vi "Get Device.vi"(6 "error in":errorcluster, 9 "String":string) -> (0 "error out 2":errorcluster, 2 "element":string, 3 "substring":string)   [LabVIEW 2013]
uses:
  <vilib>/regexp/Match Regular Expression.xnode
panel:
  out "Device Name":string
  out "Numeric":i32
  out "Sorted List":string[](array[string])
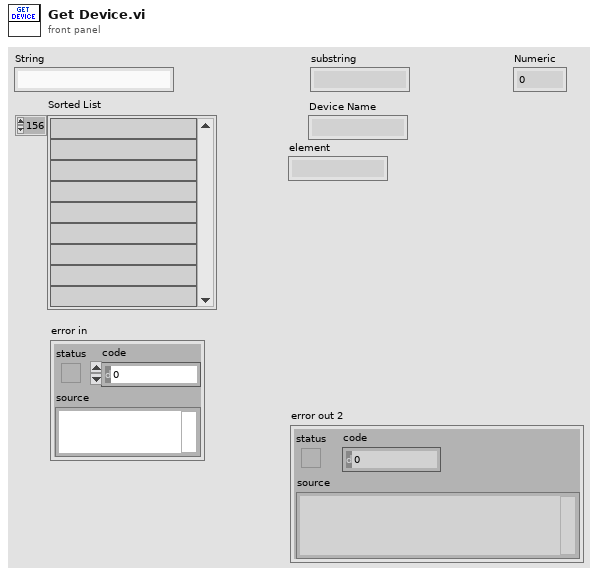
[diagram p1: front panel]
types:
  T1 = typedef "mysql_authentication.ctl" = cluster{"User":string, "Password":string, "Database":string}
  T2 = cluster{"Port":u16, "IP Address":string, "Authentication":T1}
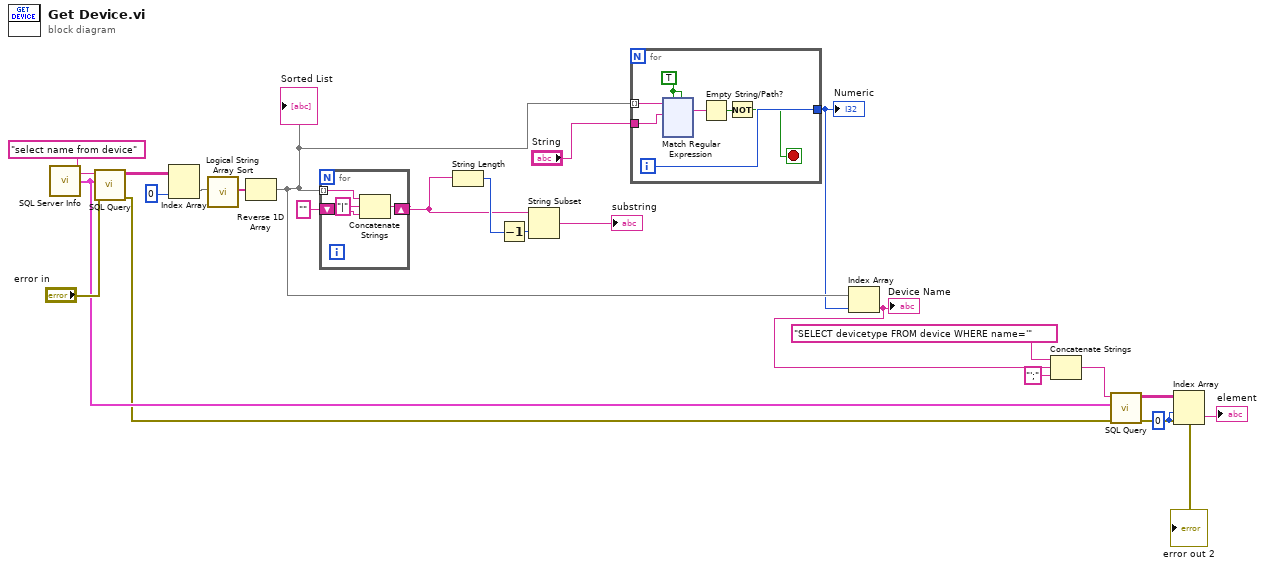
[diagram p0: block diagram]
diagram:
  w2 = 0 ("disabled index (col)")
  n1 = call "SQL Server Info.vi"() -> ("SQL Server Info"=w10:T2)
  n2 = call "SQL Query.vi"("error in (no error)"="error in", "SQL Server Info"=w10, "Query"="select name from device") -> ("error out"=w3:errorcluster, "data"=w17:string[][])  [unwired: 7 in]
  n3 = Index Array(array=w17, index (col)=0 ("disabled index (col)")) -> (element=w16:string[])  [unwired: 1 in]
  n4 = call "Logical String Array Sort.vi"("Unsorted List"=w16) -> ("Sorted List"=w15:string[])  [unwired: 18 in]
  n5 = Reverse 1D Array(array=w15) -> (reversed array=w13:string[])
  "Sorted List" <- w13
  n6 = for {
    tunnel: w13 -> [w28] mode=indexing
    shift-right: [w26] -> w23
    shift-left: "" -> [w25]
    n7 = Concatenate Strings(w28, "|" ("string"), w25) -> (w26:string)
  }
  n8 = String Length(string=w23) -> (length=w24:i32)
  n9 = Decrement(x=w24) -> (x-1=w22:i32)
  n10 = String Subset(string=w23, length (rest)=w22) -> (substring=→"substring":string)  [unwired: 1 in]
  n11 = for {
    tunnel: w13 -> [w35] mode=indexing
    tunnel: "String" -> [w34]
    tunnel: [w30] -> w12
    i -> [w30]
    stop <- w29 stop-if-true
    w33 = TRUE ("ignore case? (F)")
    n12 = xnode "Match Regular Expression"("input string"=w35, "regular expression"=w34, "ignore case? (F)"=w33, "multiline? (F)"=w33) -> ("whole match"=w32:string)  [unwired: 2 in, 4 out]
    n13 = Empty String/Path?(string/path=w32) -> (empty?=w31:bool)
    n14 = Not(x=w31) -> (.not. x?=w29:bool)
  }
  "Numeric" <- w12
  n15 = Index Array(array=w13, index=w12) -> (element=w8:string)
  "Device Name" <- w8
  n16 = Concatenate Strings("SELECT devicetype FROM device WHERE name='", w8, "';" ("string")) -> (w6:string)
  n17 = call "SQL Query.vi"("error in (no error)"=w3, "SQL Server Info"=w10, "Query"=w6) -> ("error out"=→"error out 2":errorcluster, "data"=w5:string[][])  [unwired: 7 in]
  n18 = Index Array(array=w5, index (row)=w2, index (col)=w2) -> (element=→"element":string)
